vi "Single Acquisition and RMS Test UI.vi"() -> ()   [LabVIEW 2014]
uses:
  <vilib>/rvi/interface/RandomDataEmulation/nirviRandomDataOpen.vi
  <vilib>/rvi/interface/common/niFpgaCacheSessionInfoDynamic.vi
  <vilib>/rvi/interface/common/niFpgaWaitOnOcc.vi
  <vilib>/Utility/error.llb/Error Cluster From Error Code.vi
  <vilib>/FPGAPlugInAG/Dynamic/niLvFpga_Run_Dynamic.vi
  <vilib>/rvi/errors/niLvFpgaAdjustHostInterfaceError.vi
  <vilib>/FPGAPlugInAG/Dynamic/niLvFpga_Close_Dynamic.vi
  <vilib>/rvi/interface/nirviOpenFPGA/nirviOpenFPGA.xnode
  FPGA Target/Test VIs/RMS Measurement Test.vi
  <vilib>/rvi/interface/nirviMethod/nirviMethod.xnode
  <vilib>/rvi/interface/nirviReadWriteControl/nirviReadWriteControl.xnode
  <vilib>/rvi/interface/nirviCloseFPGA/nirviCloseFPGA.xnode
  <vilib>/rvi/errors/niLvFpgaMergeErrorWithErrorCode.vi
  <vilib>/FPGAPlugInAG/Dynamic/niLvFpga_ConfigureFifo_Dynamic.vi
  <vilib>/FPGAPlugInAG/Dynamic/niLvFpga_StartFifo_Dynamic.vi
  <vilib>/FPGAPlugInAG/Dynamic/niLvFpga_ReadFifo_Dynamic.vi
  NiFpgaLv.dll
  <vilib>/rvi/interface/Simulation/niFpgaSimulationCallBeginRW.vi
panel:
  out "RMS":fxp<+,12,12>
  out "DC (Mean)":fxp<+/-,12,12>
  in  "Number of Elements to read":u32=2047
  out "Waveform Graph (input data)":dbl[](graph)
  out "Elements Remaining":u32
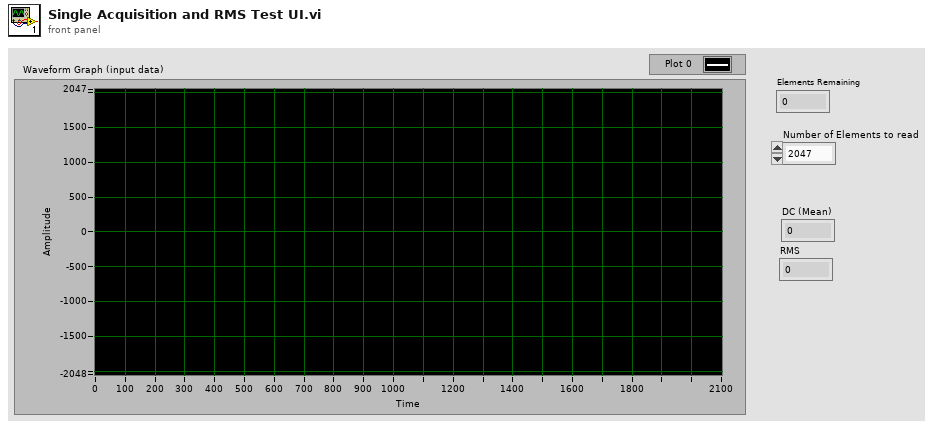
[diagram p1: front panel]
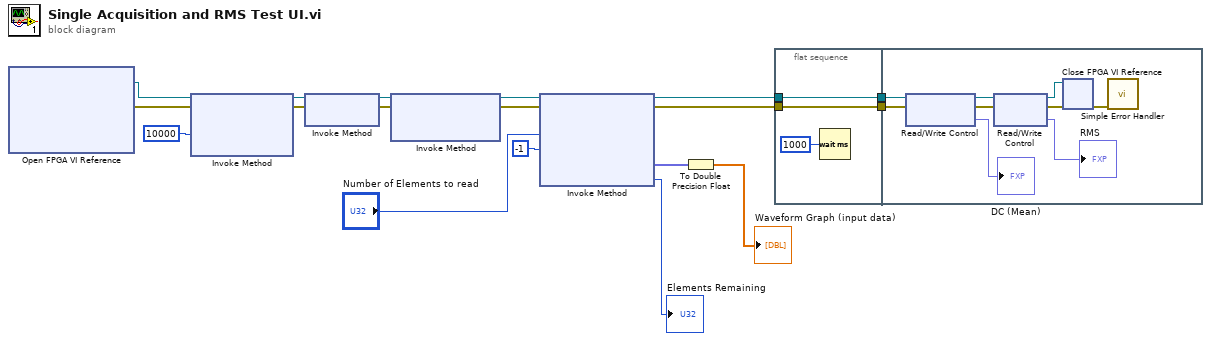
[diagram p0: block diagram]
diagram:
  n1 = xnode "Open FPGA VI Reference"() -> ("FPGA VI Reference Out"=w5:refnum<k20>, "error out"=w6:errorcluster)  [unwired: 2 in]
  n2 = xnode "Invoke Method"("FPGA VI Reference In"=w5, "error in"=w6, "Requested Depth"=u32 10000) -> ("FPGA VI Reference Out"=w16:refnum<k20>, "error out"=w17:errorcluster)  [unwired: 1 out]
  n3 = xnode "Invoke Method"("FPGA VI Reference In"=w16, "error in"=w17) -> ("FPGA VI Reference Out"=w14:refnum<k20>, "error out"=w15:errorcluster)
  n4 = xnode "Invoke Method"("FPGA VI Reference In"=w14, "error in"=w15) -> ("FPGA VI Reference Out"=w13:refnum<k20>, "error out"=w12:errorcluster)  [unwired: 1 in]
  n5 = xnode "Invoke Method"("FPGA VI Reference In"=w13, "error in"=w12, "Number of Elements"="Number of Elements to read", "Timeout (ms)"=-1) -> ("FPGA VI Reference Out"=w4:refnum<k20>, "error out"=w3:errorcluster, "Data"=w8:fxp<+/-,12,12>[], "Elements Remaining"=→"Elements Remaining":u32)
  n6 = To Double Precision Float(number=w8) -> (double precision float=→"Waveform Graph (input data)":dbl[])
  n7 = flat-sequence {
    tunnel: w3 -> [w20]
    tunnel: w4 -> [w21]
    tunnel: [w21] -> w2
    tunnel: [w20] -> w1
    tunnel: w2 -> [w27]
    tunnel: w1 -> [w26]
    frame #0 {
      n8 = Wait (ms)(milliseconds to wait=u32 1000) -> ()  [unwired: 1 out]
    }
    frame #1 {
      n9 = xnode "Read/Write Control"("FPGA VI Reference In"=w27, "error in"=w26) -> ("FPGA VI Reference Out"=w24:refnum<k20>, "error out"=w25:errorcluster, "DC (Mean)"=→"DC (Mean)":fxp<+/-,12,12>)
      n10 = xnode "Read/Write Control"("FPGA VI Reference In"=w24, "error in"=w25) -> ("FPGA VI Reference Out"=w23:refnum<k20>, "error out"=w22:errorcluster, "RMS"=→"RMS":fxp<+,12,12>)
      n11 = xnode "Close FPGA VI Reference"("FPGA VI Reference In"=w23, "error in"=w22) -> ("error out"=w28:errorcluster)
      n12 = call <vilib>:"Simple Error Handler.vi"("error in (no error)"=w28) -> ()  [unwired: 4 in, 5 out]
    }
  }
